vi "Temp & Vol.vi"() -> (0 "温度":dbl(slide) scale=0.0..100.0, 1 "容积":dbl(slide) scale=0.0..1000.0)   [LabVIEW 2010]
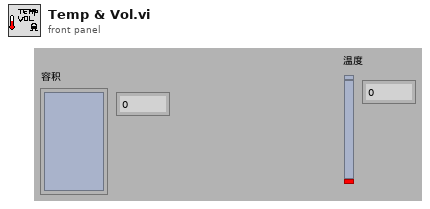
[diagram p1: front panel]
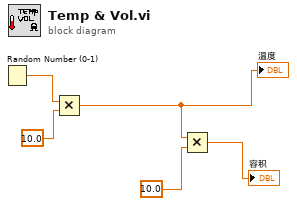
[diagram p0: block diagram]
diagram:
  n1 = Random Number (0-1)() -> (number: 0 to 1=w5:dbl)
  n2 = Multiply(x=w5, y=10.0) -> (x*y=w2:dbl)
  "温度" <- w2
  n3 = Multiply(x=w2, y=10.0) -> (x*y=→"容积":dbl)
